vi "HW2.vi"() -> ()   [LabVIEW 2021]
panel:
  in  "Send value 7":dbl
  in  "Send value 1":dbl
  in  "Send value 8":dbl
  in  "Send value 6":dbl
  in  "Send value 5":dbl
  in  "Send value 4":dbl
  in  "Send value 3":dbl
  in  "Send value 2":dbl
  in  "Send button":bool
  out "RecvValue 8":dbl
  out "RecvValue 7":dbl
  out "RecvValue 6":dbl
  out "RecvValue 5":dbl
  out "RecvValue 4":dbl
  out "RecvValue 3":dbl
  out "Y":dbl
  out "X":dbl
  in  "Display History":bool
  in  "Size of Rectangle":i16=20
  in  "stop":bool
  out "2D Picture":picture
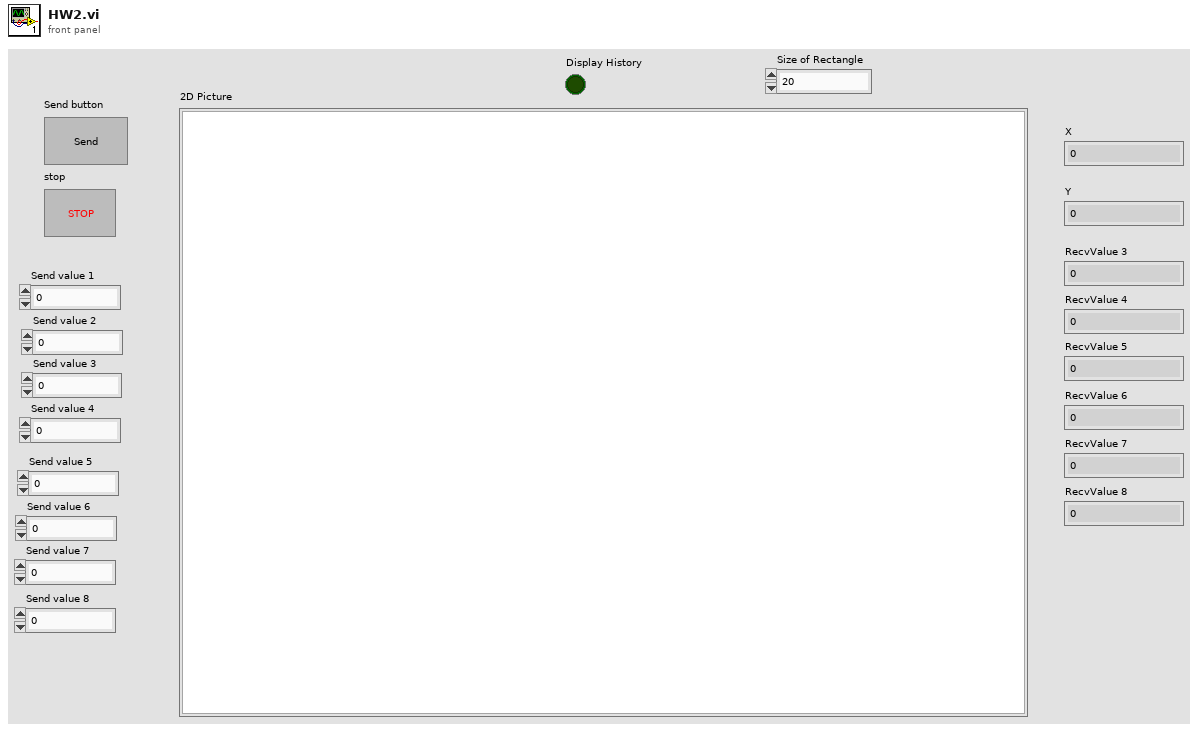
[diagram p1: front panel]
types:
  T1 = enum16{"Standard", "Buffered", "CRLF", "Immediate"}
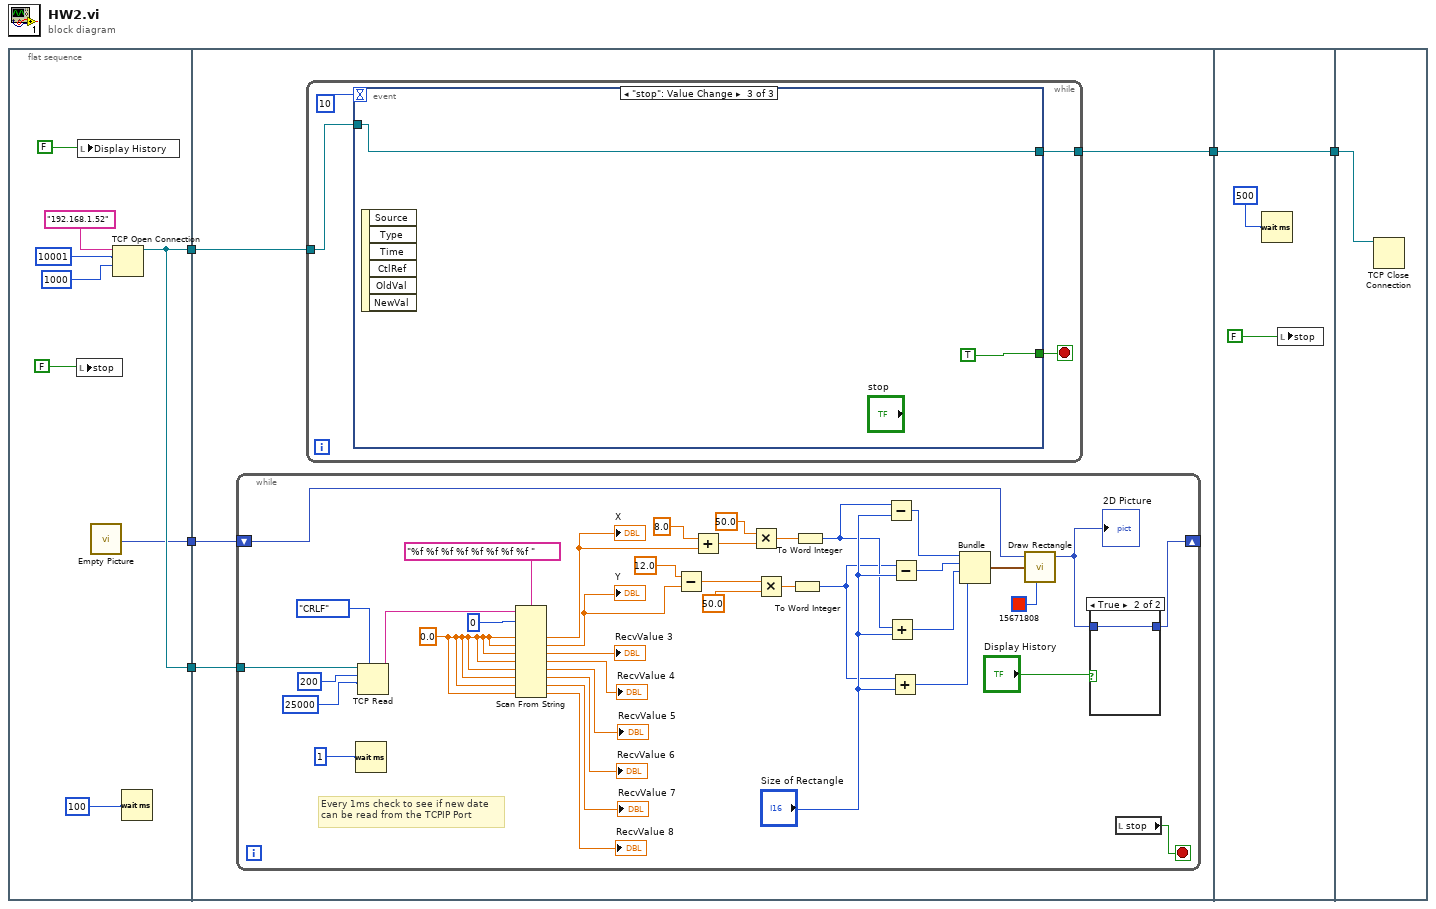
[diagram p0: block diagram]
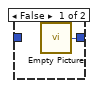
[diagram p2: hidden frame]
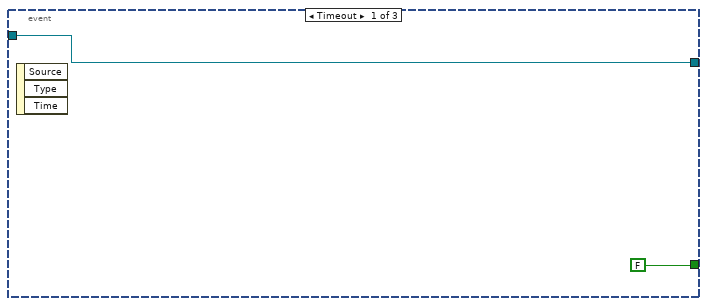
[diagram p3: hidden frame]
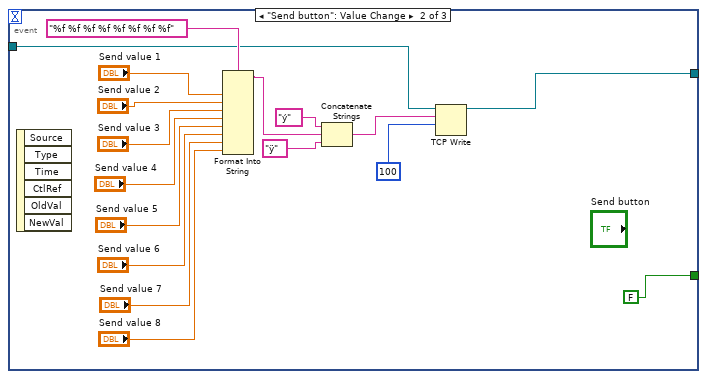
[diagram p4: hidden frame]
diagram:
  n1 = flat-sequence {
    tunnel: [w9] -> w5
    tunnel: [w9] -> w2
    tunnel: [w8] -> w1
    tunnel: w5 -> [w17]
    tunnel: [w16] -> w3
    tunnel: w2 -> [w15]
    tunnel: w1 -> [w14]
    tunnel: [w86] -> w4
    tunnel: w3 -> [w86]
    tunnel: w4 -> [w87]
    frame #0 {
      n2 = local write "stop"(FALSE) -> ()
      n3 = local write "Display History"(FALSE) -> ()
      n4 = call "Empty Picture"() -> ("empty picture"=w8:picture)
      n5 = TCP Open Connection(address="192.168.1.52", remote port or service name=u16 10001, timeout ms (60000)=1000) -> (connection ID=w9:refnum<k5>)  [unwired: 2 in, 1 out]
      n6 = Wait (ms)(milliseconds to wait=u32 100) -> ()  [unwired: 1 out]
    }
    frame #1 {
      n7 = while {
        tunnel: w15 -> [w55]
        shift-right: [w22] -> _
        shift-left: w14 -> [w21]
        stop <- w19 stop-if-true
        w50 = 0.0 ("default value 1")
        # "Every 1ms check to see if new date\ncan be read from the TCPIP Port"
        n8 = Wait (ms)(milliseconds to wait=u32 1) -> ()  [unwired: 1 out]
        n9 = TCP Read(connection ID=w55, bytes to read=200, 7:T1."CRLF" ("mode (standard)"), 9:25000 ("timeout ms (25000)")) -> (data out=w51:string)  [unwired: 1 in, 2 out]
        n10 = Scan From String "Scan From String"(format string="%f %f %f %f %f %f %f %f ", input string=w51, initial scan location=u32 0, default 1=w50, default 2=w50, default 3=w50, default 4=w50, default 5=w50, default 6=w50, default 7=w50, default 8=w50) -> (output 1=w41:dbl, output 2=w39:dbl, output 3=→"RecvValue 3":dbl, output 4=→"RecvValue 4":dbl, output 5=→"RecvValue 5":dbl, output 6=→"RecvValue 6":dbl, output 7=→"RecvValue 7":dbl, output 8=→"RecvValue 8":dbl)  [unwired: 1 in, 3 out]
        "X" <- w41
        "Y" <- w39
        n11 = Subtract(x=12.0, y=w39) -> (x-y=w35:dbl)
        n12 = Add(x=8.0, y=w41) -> (x+y=w34:dbl)
        n13 = Multiply(x=50.0, y=w34) -> (x*y=w38:dbl)
        n14 = Multiply(x=w35, y=50.0) -> (x*y=w37:dbl)
        n15 = To Word Integer(number=w37) -> (16bit integer=w30:i16)
        n16 = To Word Integer(number=w38) -> (16bit integer=w31:i16)
        n17 = Subtract(x=w31, y="Size of Rectangle") -> (x-y=w29:i16)
        n18 = Add(x=w31, y="Size of Rectangle") -> (x+y=w27:i16)
        n19 = Add(x=w30, y="Size of Rectangle") -> (x+y=w26:i16)
        n20 = Subtract(x=w30, y="Size of Rectangle") -> (x-y=w28:i16)
        n21 = Bundle(w29, w28, w27, w26) -> (w25:cluster{i16, i16, i16, i16})  [unwired: 1 in]
        n22 = call <vilib>:"Draw Rectangle.vi"("picture"=w21, "rect"=w25, "color(black)"=u32 15671808) -> ("new picture"=w23:picture)  [unwired: 6 in]
        "2D Picture" <- w23
        n23 = case shown="True" "Display History" {
          tunnel: [w57 w58] -> w22
          tunnel: w23 -> [_ w58]
          frame False {
            n24 = call "Empty Picture"() -> ("empty picture"=w57:picture)
          }
          frame True {
          }
        }
        n25 = local read "stop"() -> (w19:bool)
      }
      n26 = while {
        tunnel: w17 -> [w61]
        tunnel: [w59] -> w16
        stop <- w60 stop-if-true
        n27 = event shown="[2] \"stop\": Value Change" {
          selector: _ -> [_ _ _]
          dyn-events: _ -> [_ _ _]
          timeout: 10 -> [_ _ _]
          tunnel: w61 -> [w63 w66 w82]
          tunnel: [FALSE FALSE TRUE] -> w60
          tunnel: [w63 w65 w82] -> w59
          event Timeout {
            n28 = event-data() -> ()  [unwired: 1 in, 3 out]
          }
          event "Send button": Value Change {
            n29 = event-data() -> ()  [unwired: 1 in, 6 out]
            n30 = Format Into String "Format Into String"(format string="%f %f %f %f %f %f %f %f", "Send value 1", "Send value 2", "Send value 3", "Send value 4", "Send value 5", "Send value 6", "Send value 7", "Send value 8") -> (resulting string=w73:string)  [unwired: 2 in, 1 out]
            n31 = Concatenate Strings("ý" ("string"), w73, "ÿ" ("string")) -> (w67:string)
            n32 = TCP Write(connection ID=w66, data in=w67, 9:100 ("timeout ms (25000)")) -> (connection ID out=w65:refnum<k5>)  [unwired: 1 in, 2 out]
          }
          event "stop": Value Change {
            n33 = event-data() -> ()  [unwired: 1 in, 6 out]
          }
        }
      }
    }
    frame #2 {
      n34 = Wait (ms)(milliseconds to wait=u32 500) -> ()  [unwired: 1 out]
      n35 = local write "stop"(FALSE) -> ()
    }
    frame #3 {
      n36 = TCP Close Connection(connection ID=w87) -> ()  [unwired: 2 in, 2 out]
    }
  }
